vi "picoquant_initialize_acq_mode.vi"(8 "error in (no error)":errorcluster, 11 "picoharp in":refnum<class "picoharp.lvclass">) -> (0 "error out":errorcluster, 3 "picoharp out":refnum<class "picoharp.lvclass">)   [LabVIEW 2015, in "picoharp.lvclass"]
uses:
  picoharp.lvclass
  picoharp.lvclass/picoharp.ctl
  phlib.dll
panel:
  out "version":u8[](array[numeric])
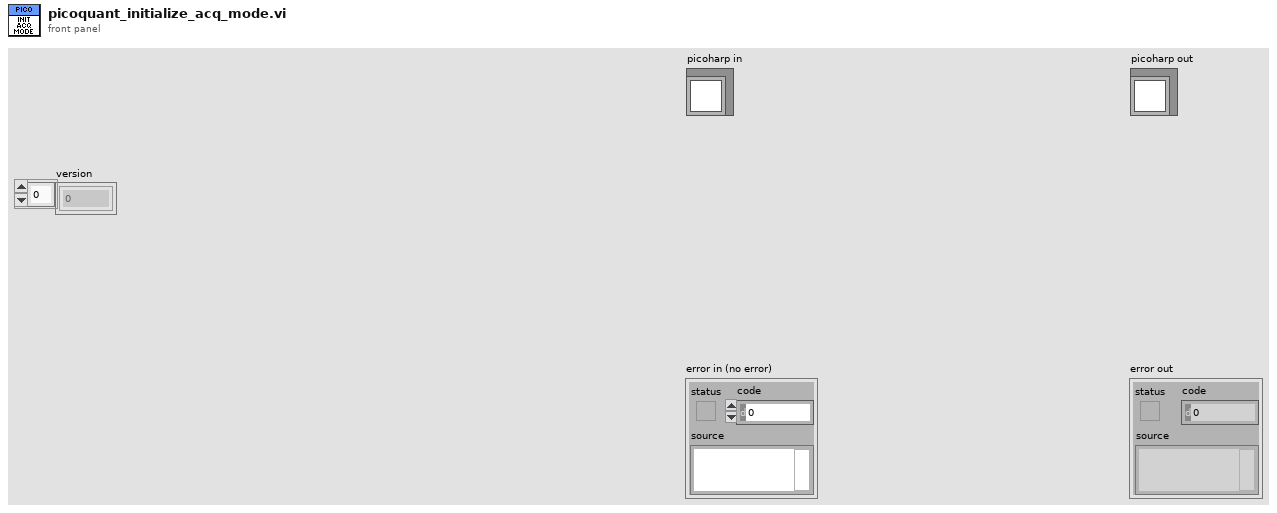
[diagram p1: front panel]
types:
  T1 = typedef "hpanel_acq_modes.ctl" = u16
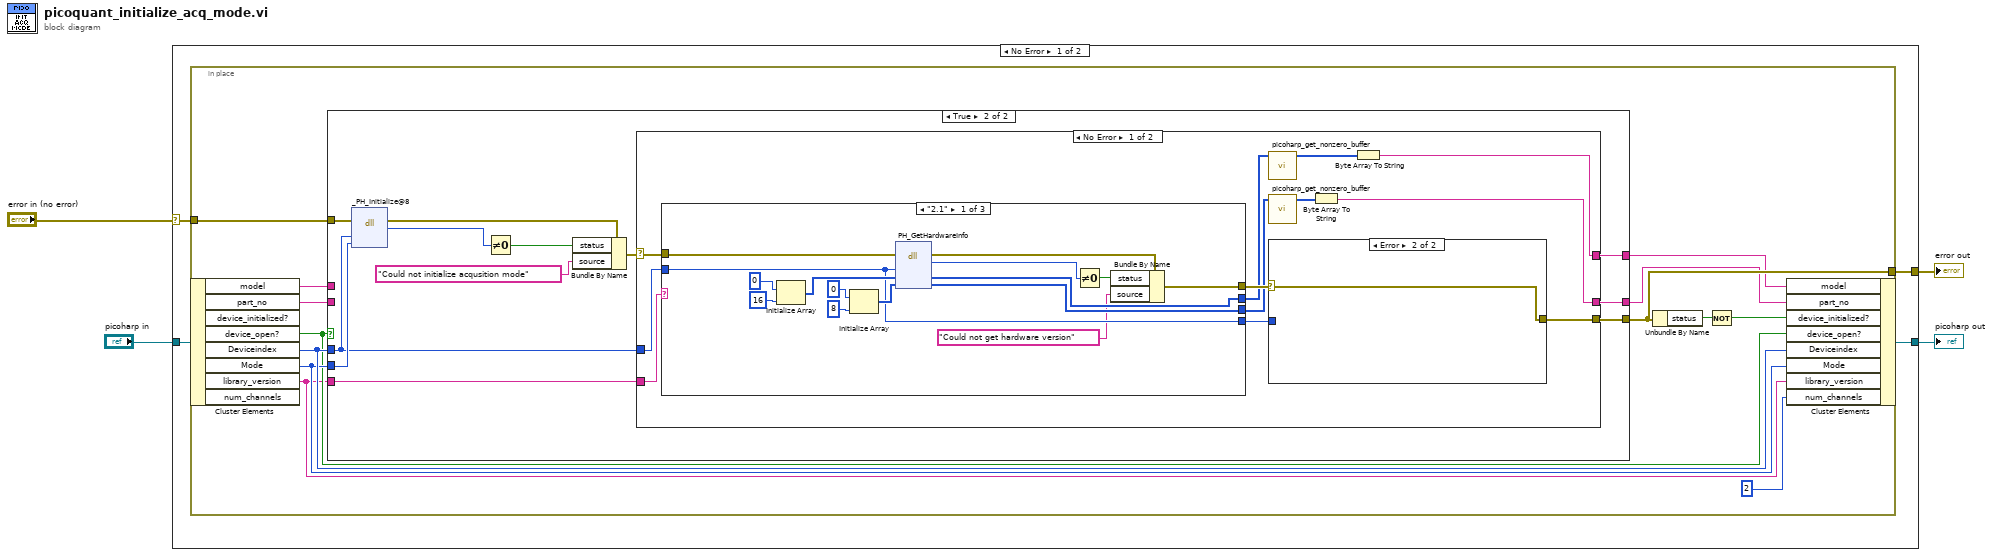
[diagram p0: block diagram]
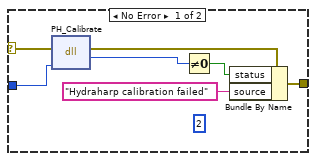
[diagram p3: hidden frame]
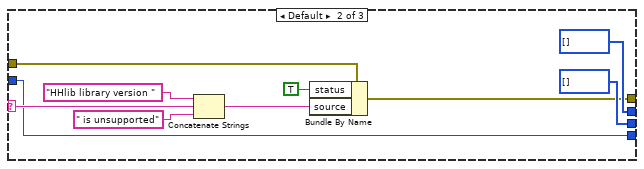
[diagram p4: hidden frame]
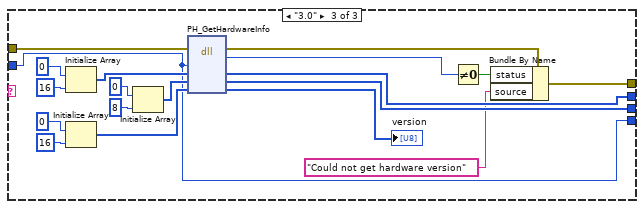
[diagram p5: hidden frame]
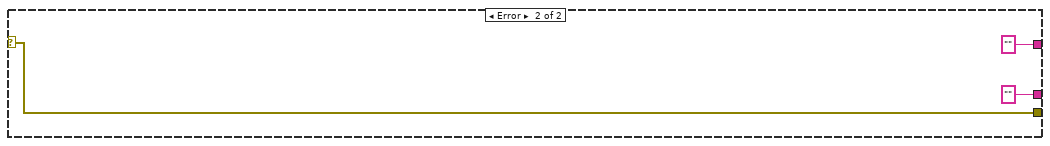
[diagram p6: hidden frame]
diagram:
  n1 = case shown="No Error" "error in (no error)" {
    selector: "error in (no error)" -> [w7 w105]
    tunnel: [w6 w105] -> w1
    tunnel: [w5 w104] -> w2
    tunnel: "picoharp in" -> [w8 w104]
    frame No Error {
      n2 = in-place {
        in-place-border: w7 -> [w21]
        in-place-border: [w17] -> w6
        n3 = in-place-cluster #1(w8) -> ("model"=w12:string, "part_no"=w11:string, "device_open?"=w18:bool, "Deviceindex"=w20:i32, "Mode"=w19:T1, "library_version"=w10:string)  [unwired: 2 out]
        n4 = case shown="True" w18 {
          tunnel: w21 -> [w24 w36]
          tunnel: [w24 w34] -> w17
          tunnel: w20 -> [_ w33]
          tunnel: w19 -> [_ w35]
          tunnel: [w23 w32] -> w14
          tunnel: [w22 w31] -> w13
          tunnel: w12 -> [w23 _]
          tunnel: w11 -> [w22 _]
          tunnel: w10 -> [_ w30]
          frame False {
          }
          frame True {
            n5 = dll-call lib="phlib.dll" fn="_PH_Initialize@8"(error in=w36, "devidx"=w33, "mode"=w35) -> (error out=w28:errorcluster, "return type"=w29:i32)  [unwired: 4 in, 1 out]
            n6 = Not Equal To 0?(x=w29) -> (x != 0?=w27:bool)
            n7 = Bundle By Name(cluster=w28, "status"=w27, "source"="Could not initialize acqusition mode") -> (w25:errorcluster)
            n8 = case shown="No Error" w25 {
              selector: w25 -> [w38 w101]
              tunnel: [w37 w101] -> w34
              tunnel: w33 -> [w48 _]
              tunnel: [w42 "" ("string")] -> w32
              tunnel: [w41 "" ("string")] -> w31
              tunnel: w30 -> [w40 _]
              frame No Error {
                n9 = case shown="\"2.1\"" w40 {
                  selector: w40 -> [_ w78 _]
                  tunnel: w38 -> [w71 w76 w100]
                  tunnel: w48 -> [w62 w72 w87]
                  tunnel: [w59 w75 w82] -> w47
                  tunnel: [w64 u8[] [] ("Model") w93] -> w46
                  tunnel: [w63 u8[] [] ("Partno") w92] -> w45
                  tunnel: [w62 w72 w87] -> w39
                  frame "2.1" {
                    n10 = Initialize Array(u8 0 ("element"), 16 ("dimension size")) -> (w68:u8[])
                    n11 = Initialize Array(u8 0 ("element"), 8 ("dimension size")) -> (w65:u8[])
                    n12 = dll-call lib="phlib.dll" fn="PH_GetHardwareInfo" label="HH_GetHardwareVersion"(error in=w71, "devidx"=w62, "Model"=w68, "Partno"=w65) -> (error out=w60:errorcluster, "return type"=w58:i32, "Model"=w64:u8[], "Partno"=w63:u8[])  [unwired: 3 in, 1 out]
                    n13 = Not Equal To 0?(x=w58) -> (x != 0?=w57:bool)
                    n14 = Bundle By Name(cluster=w60, "status"=w57, "source"="Could not get hardware version") -> (w59:errorcluster)
                  }
                  frame Default {
                    n15 = Concatenate Strings("HHlib library version " ("string"), w78, " is unsupported" ("string")) -> (w73:string)
                    n16 = Bundle By Name(cluster=w76, "status"=TRUE, "source"=w73) -> (w75:errorcluster)
                  }
                  frame "3.0" {
                    n17 = Initialize Array(u8 0 ("element"), 16 ("dimension size")) -> (w97:u8[])
                    n18 = Initialize Array(u8 0 ("element"), 16 ("dimension size")) -> (w89:u8[])
                    n19 = Initialize Array(u8 0 ("element"), 8 ("dimension size")) -> (w94:u8[])
                    n20 = dll-call lib="phlib.dll" fn="PH_GetHardwareInfo" label="HH_GetHardwareVersion"(error in=w100, "devidx"=w87, "Model"=w97, "Partno"=w94, "version"=w89) -> (error out=w85:errorcluster, "return type"=w86:i32, "Model"=w93:u8[], "Partno"=w92:u8[], "version"=→"version":u8[])  [unwired: 3 in, 1 out]
                    n21 = Not Equal To 0?(x=w86) -> (x != 0?=w84:bool)
                    n22 = Bundle By Name(cluster=w85, "status"=w84, "source"="Could not get hardware version") -> (w82:errorcluster)
                  }
                }
                n23 = call "picoharp_get_nonzero_buffer.vi"("buffer"=w46) -> ("subarray"=w43:u8[])  [unwired: 10 in]
                n24 = call "picoharp_get_nonzero_buffer.vi"("buffer"=w45) -> ("subarray"=w44:u8[])  [unwired: 10 in]
                n25 = case shown="Error" w47 {
                  selector: w47 -> [w55 w56]
                  tunnel: w39 -> [w49 _]
                  tunnel: [w52 w56] -> w37
                  frame No Error {
                    (unwired) 2 ("num_channels")
                    n26 = dll-call lib="phlib.dll" fn="PH_Calibrate"(error in=w55, "devidx"=w49) -> (error out=w53:errorcluster, "return type"=w54:i32)  [unwired: 3 in, 1 out]
                    n27 = Not Equal To 0?(x=w54) -> (x != 0?=w51:bool)
                    n28 = Bundle By Name(cluster=w53, "status"=w51, "source"="Hydraharp calibration failed") -> (w52:errorcluster)
                  }
                  frame Error {
                  }
                }
                n29 = Byte Array To String(unsigned byte array=w44) -> (string=w41:string)
                n30 = Byte Array To String(unsigned byte array=w43) -> (string=w42:string)
              }
              frame Error {
              }
            }
          }
        }
        n31 = Unbundle By Name(w17) -> ("status"=w16:bool)
        n32 = Not(x=w16) -> (.not. x?=w15:bool)
        n33 = in-place-cluster #1("model"=w14, "part_no"=w13, "device_initialized?"=w15, "device_open?"=w18, "Deviceindex"=w20, "Mode"=w19, "library_version"=w10, "num_channels"=2) -> (w5:refnum<class "picoharp.lvclass">)
      }
    }
    frame Error {
    }
  }
  "error out" <- w1
  "picoharp out" <- w2
